vi "Set Title.vi"(8 "error in (no error)":errorcluster, 10 "title":string, 11 "UI_ProgressBar in":refnum<class "UI_ProgressDlg.lvclass">) -> (0 "error out":errorcluster, 3 "UI_ProgressBar out":refnum<class "UI_ProgressDlg.lvclass">)   [LabVIEW 2014, in "UI_ProgressDlg.lvlib" / "UI_ProgressDlg.lvclass"]
uses:
  UI_ProgressDlg.lvclass
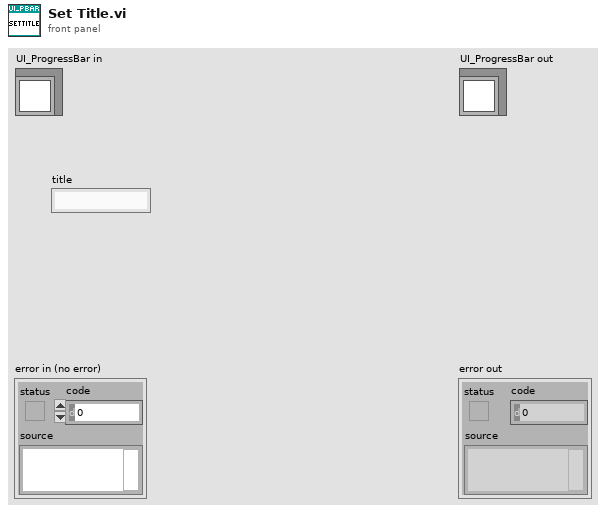
[diagram p1: front panel]
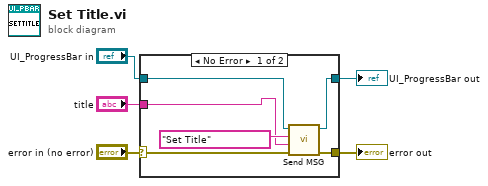
[diagram p0: block diagram]
diagram:
  n1 = case shown="No Error" "error in (no error)" {
    selector: "error in (no error)" -> [w11 w13]
    tunnel: [w9 w13] -> w4
    tunnel: [w8 w12] -> w2
    tunnel: "UI_ProgressBar in" -> [w10 w12]
    tunnel: "title" -> [w6 _]
    frame No Error {
      n2 = call "Send MSG.vi"("error in (no error)"=w11, "msg value"=w6, "msg"="Set Title" ("Inforamtion"), "UI_ProgressBar in"=w10) -> ("error out"=w9:errorcluster, "UI_ProgressBar out"=w8:refnum<class "UI_ProgressDlg.lvclass">)  [unwired: 6 in]
    }
    frame Error {
    }
  }
  "error out" <- w4
  "UI_ProgressBar out" <- w2
